vi "Servo MSMT Get ET Timing Search Step from DB.vi"(8 "error in (no error)":errorcluster, 11 "Servo MSMT in":refnum<class "Servo MSMT.lvclass">) -> (0 "error out":errorcluster, 2 "Step Out":refnum<k7>, 3 "Servo MSMT out":refnum<class "Servo MSMT.lvclass">)   [LabVIEW 2014, in "Servo MSMT.lvclass"]
uses:
  Servo MSMT.lvclass
  QPA Measurement/QPA Measurement.lvlibp/Sequence Automation/Classes/QPA Measurement/Protected Methods/Read Measurement Name.vi
  QPA Measurement/QPA Measurement.lvlibp/Sequence Automation/Classes/QPA Measurement/QPA Measurement.lvclass
  TestStand API Tools/Step Actions/TSAT Step Actions.lvlib
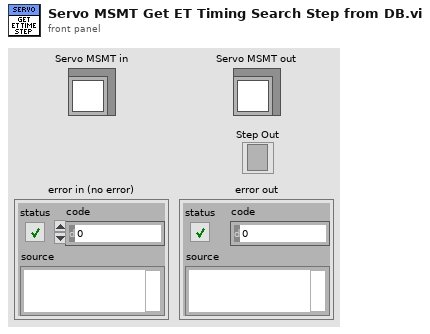
[diagram p1: front panel]
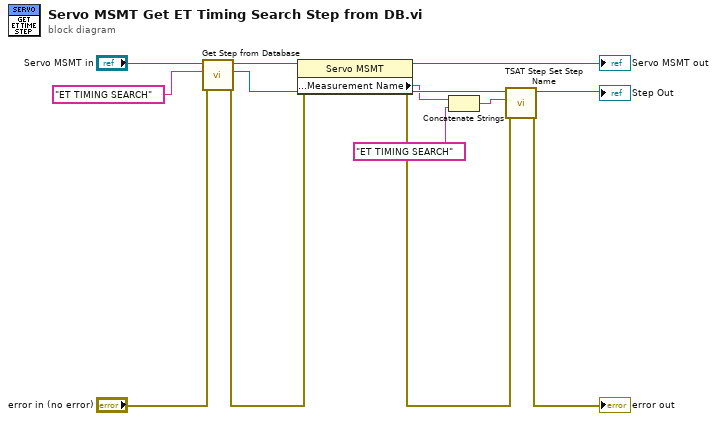
[diagram p0: block diagram]
diagram:
  n1 = call "Get Step from Database.vi"("error in (no error)"="error in (no error)", "Default Step"="ET TIMING SEARCH", "QPA Measurement in"="Servo MSMT in") -> ("error out"=w10:errorcluster, "Step Out"=w13:refnum<k7>, "QPA Measurement out"=w8:refnum<class "Servo MSMT.lvclass">)  [unwired: 6 in]
  n2 = property class="Servo MSMT"(reference=w8, error in=w10) -> (reference out=→"Servo MSMT out":refnum<class "Servo MSMT.lvclass">, error out=w9:errorcluster, "Protected Methods:Measurement Name"=w6:string)
  n3 = Concatenate Strings(w6, "ET TIMING SEARCH" ("string")) -> (w5:string)
  n4 = call "TSAT Step Set Step Name.vi"("Error In"=w9, "Name"=w5, "Step In"=w13) -> ("Error Out"=→"error out":errorcluster, "Step Out"=→"Step Out":refnum<k7>)  [unwired: 7 in]
